vi "nanoVoltRead_Lock-In.vi"() -> ()   [LabVIEW 2014]
uses:
  <vilib>/Utility/file.llb/Write To Spreadsheet File (string).vi
  subvi/Stanford Research 830/Stanford Research 830.lvlib
panel:
  in  "Boolean":bool
  in  "Ref Freq (Hz)":dbl=17.0
  in  "Phase":dbl
  out "Voltage Setpoint (V)":dbl
  in  "VISA resource name":refnum<visa-resource-name>="GPIB0::8::INSTR"
  in  "Time2\n(s)":dbl[](array[numeric])
  in  "Voltage\n(V)":dbl[](array[numeric])
  in  "Filename Label (optional)":string
  in  "Channel\n(0,1,2)":dbl[](array[numeric])
  out "Light Intensity":dbl
  in  "Time1\n(s)":dbl[](array[numeric])
  in  "Intensity\n(0-100%)":dbl[](array[numeric])
  in  "Baud Rate":dbl=57600.0
  in  "Light Port":refnum<visa-resource-name>="COM4"
  in  "Previous Top T":dbl
  in  "Temp Rate (s)":dbl=0.25
  in  "Previous Delta T":dbl
  in  "T read time":dbl
  out "Temp2 (C)":dbl format="%#.4g"
  out "Temp1 (C)":dbl format="%#.4g"
  out "Delta T (C)":dbl format="%#.4g"
  in  "Temp2 Port":tag="Dev2"
  in  "Temp1 Port":tag="Dev1"
  out "Time (s)":dbl caption="Elapsed Time (s)"
  out "XY Graph":cluster{dbl[], dbl[]}[](graph)
  in  "file (use dialog)":path=path "C:/Users/probe_station/Desktop/nanoVolt"
  out "Measurement Number":i32
  in  "stop":bool
  out "Voltage(uV)":dbl
  # "SR830\n2016-01-20\nDavid Ellsworth\nCSU Magnetics Lab"
  # "Ignore These"
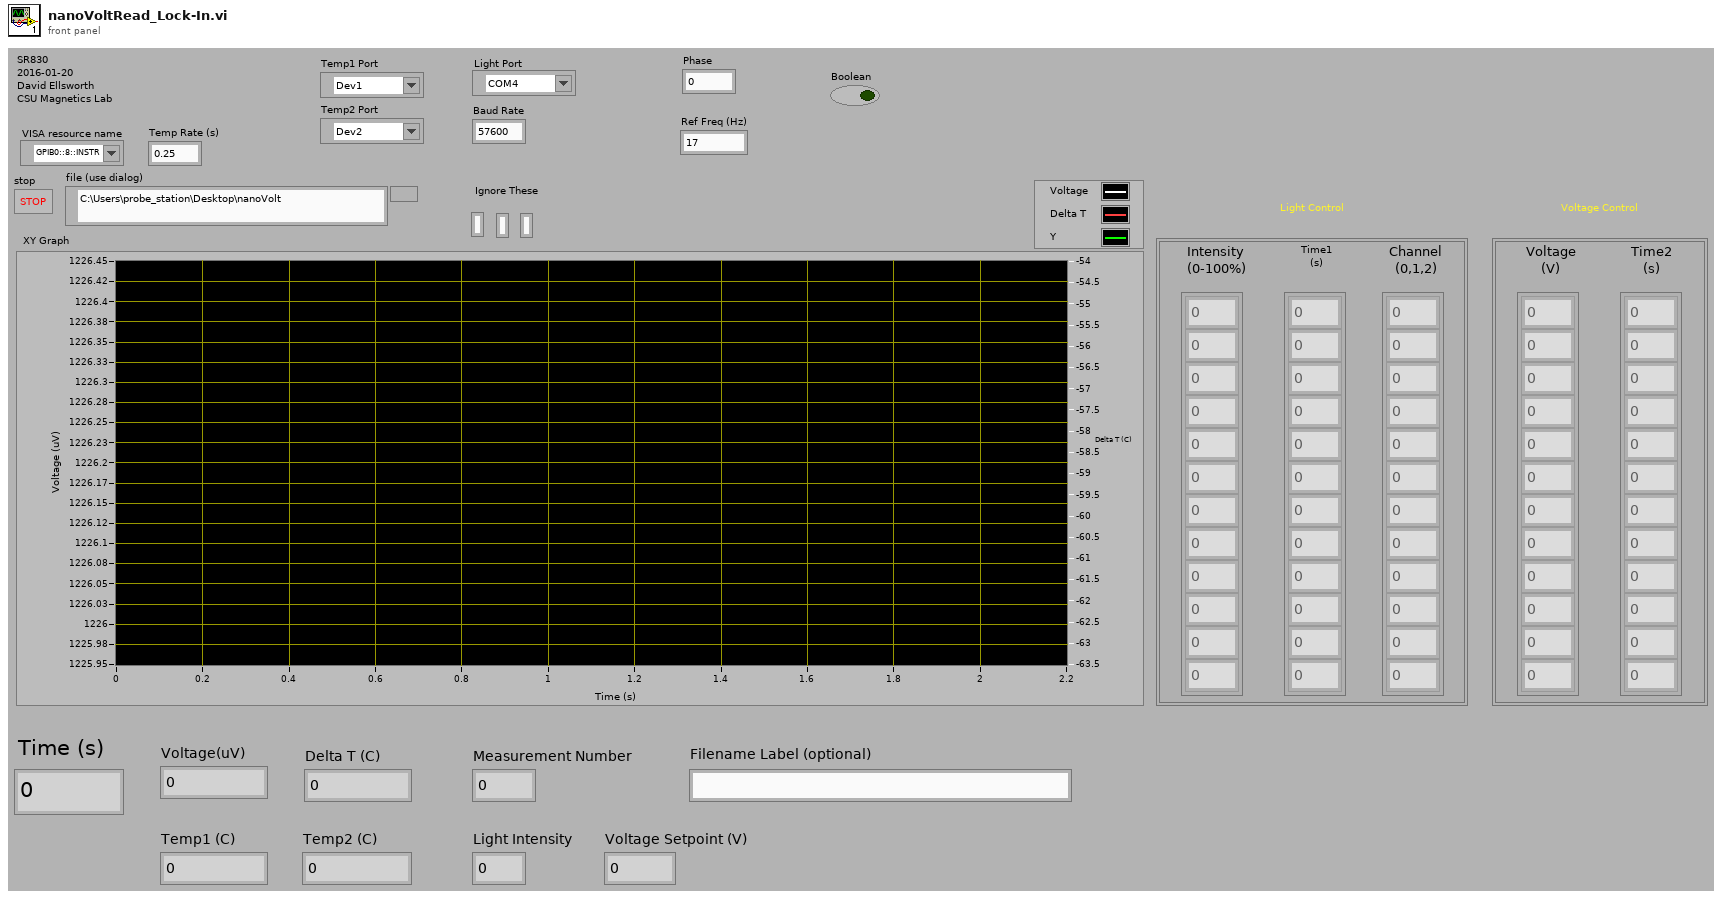
[diagram p1: front panel]
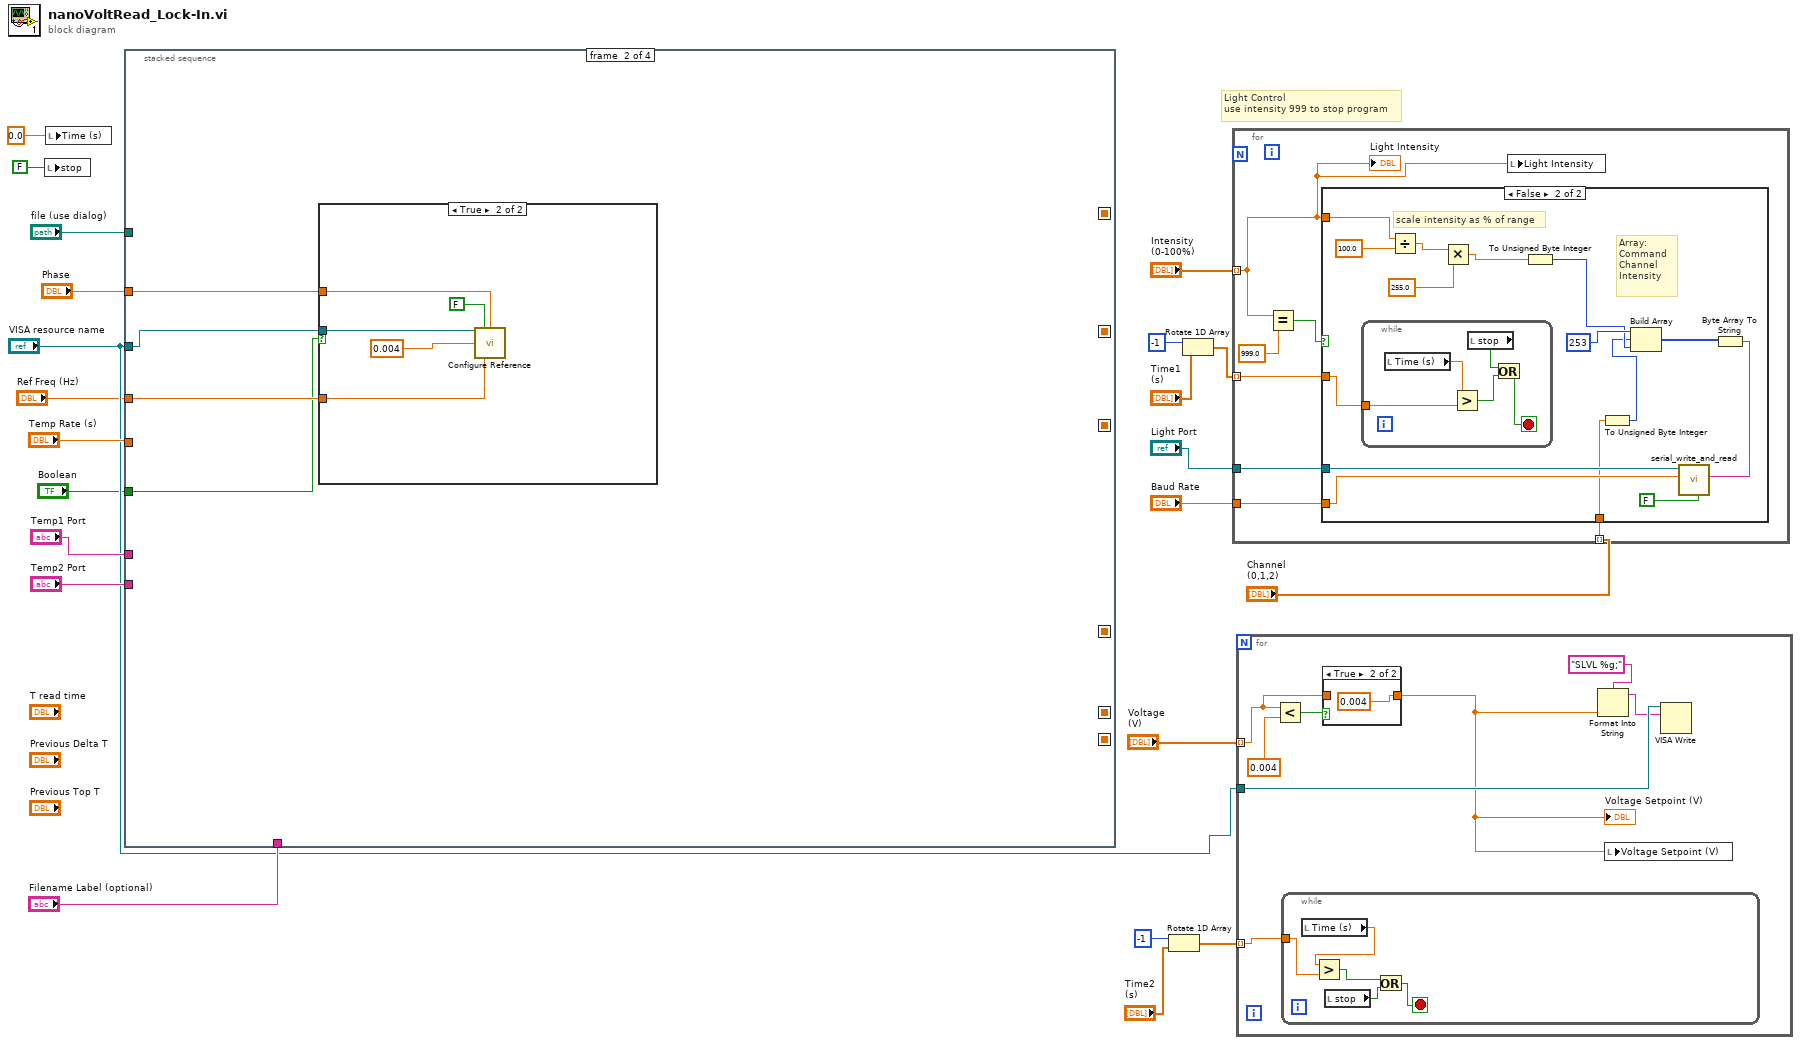
[diagram p0: block diagram]
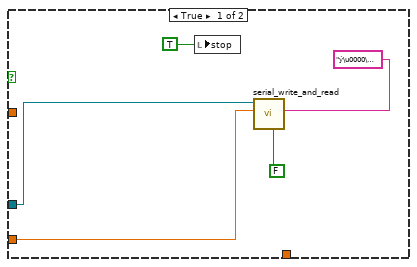
[diagram p3: hidden frame]
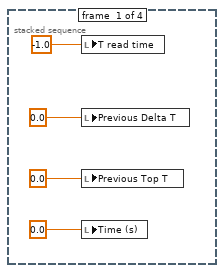
[diagram p4: hidden frame]
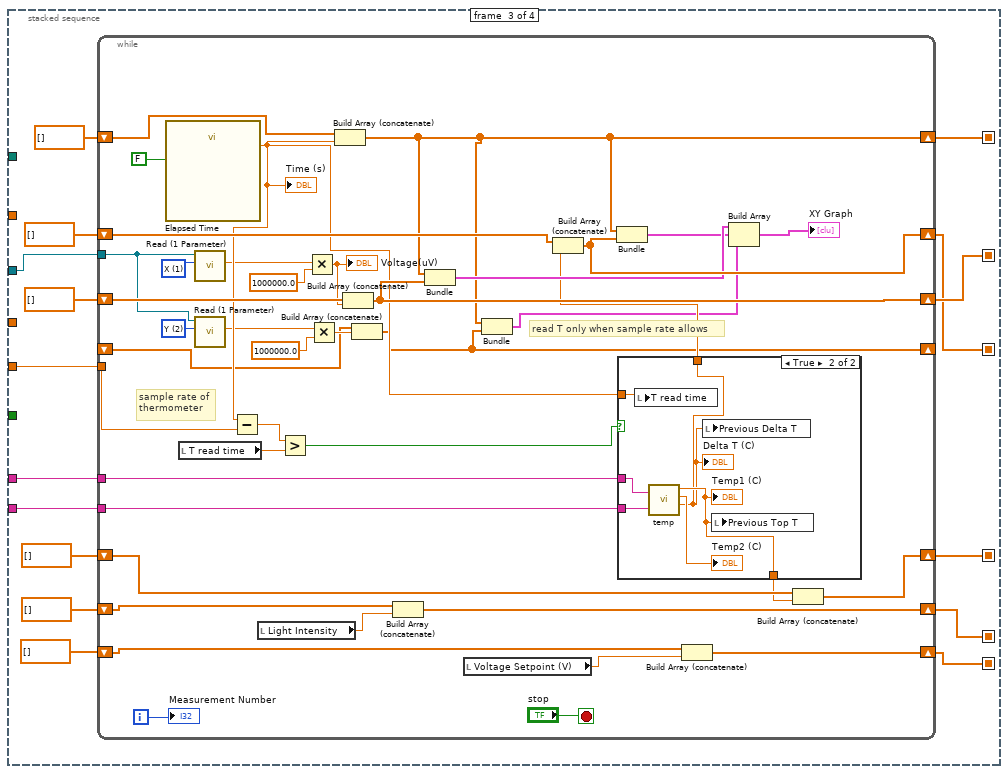
[diagram p6: hidden frame]
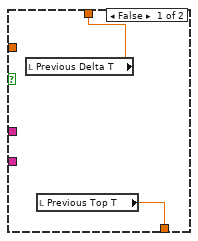
[diagram p7: hidden frame]
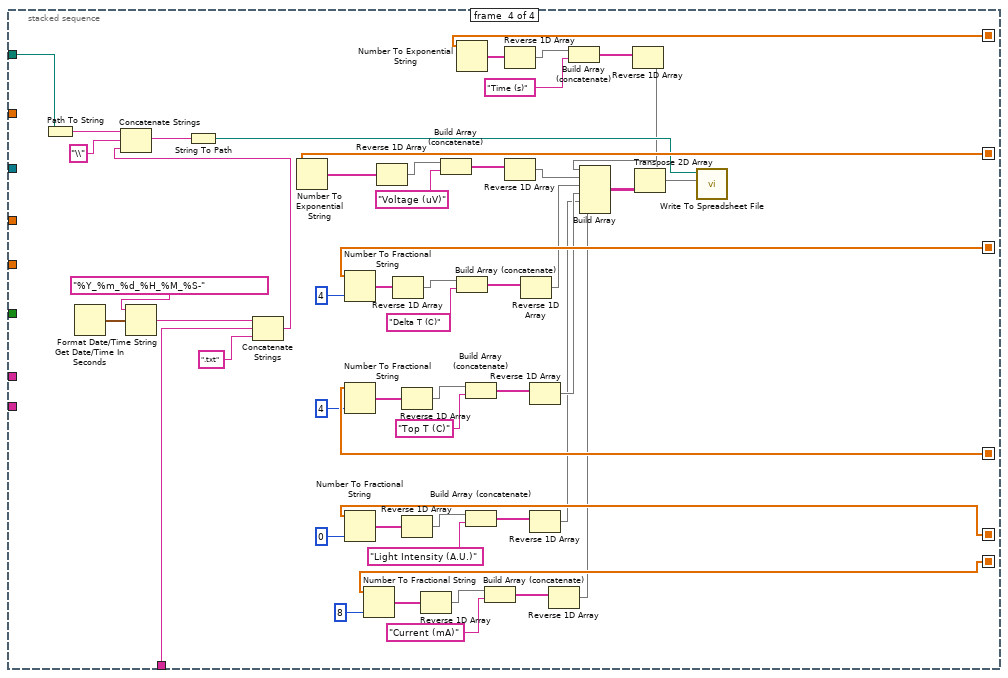
[diagram p8: hidden frame]
diagram:
  # "Light Control\nuse intensity 999 to stop program"
  n1 = local write "stop"(FALSE ("stop")) -> ()
  n2 = local write "Time (s)"(0.0 ("Time (s)")) -> ()
  n3 = stacked-sequence {
    seq-local: [_ _ w50 _] -> [_ _ _ w145]
    seq-local: [_ _ w48 _] -> [_ _ _ w138]
    seq-local: [_ _ w45 _] -> [_ _ _ w142]
    seq-local: [_ _ w42 _] -> [_ _ _ w140]
    seq-local: [_ _ w39 _] -> [_ _ _ w111]
    seq-local: [_ _ w37 _] -> [_ _ _ w102]
    tunnel: "file (use dialog)" -> [_ _ _ w147]
    tunnel: "Temp1 Port" -> [_ _ w47 _]
    tunnel: "Temp2 Port" -> [_ _ w46 _]
    tunnel: "Temp Rate (s)" -> [_ _ w43 _]
    tunnel: "Filename Label (optional)" -> [_ _ _ w108]
    tunnel: "VISA resource name" -> [_ w30 w36 _]
    tunnel: "Phase" -> [_ w29 _ _]
    tunnel: "Ref Freq (Hz)" -> [_ w28 _ _]
    tunnel: "Boolean" -> [_ w27 _ _]
    frame #0 {
      n4 = local write "T read time"(-1.0 ("read T")) -> ()
      n5 = local write "Previous Delta T"(0.0 ("Previous T")) -> ()
      n6 = local write "Previous Top T"(0.0 ("Previous Top T")) -> ()
      n7 = local write "Time (s)"(0.0 ("Time (s)")) -> ()
    }
    frame #1 {
      n8 = case shown="True" w27 {
        tunnel: w30 -> [_ w35]
        tunnel: w29 -> [_ w32]
        tunnel: w28 -> [_ w31]
        frame False {
        }
        frame True {
          n9 = call "Configure Reference.vi"("VISA resource name"=w35, "Auto Phase (T: Enabled)"=FALSE, "Manual Phase (0 Degree)"=w32, "Sine Output Amplitude (1 V)"=0.004, "Internal Reference Frequency (1000 Hz)"=w31) -> ()  [unwired: 9 in, 2 out]
        }
      }
    }
    frame #2 {
      n10 = while {
        shift-right: [w91] -> w50
        shift-left: dbl[] [] -> [w90]
        shift-right: [w54] -> w48
        shift-left: dbl[] [] -> [w88]
        tunnel: w47 -> [w87]
        tunnel: w46 -> [w86]
        shift-right: [w85] -> w45
        shift-left: dbl[] [] -> [w84]
        tunnel: w43 -> [w83]
        shift-right: [w81] -> w42
        shift-left: dbl[] [] -> [w82]
        shift-right: [w79] -> w39
        shift-left: dbl[] [] -> [w80]
        shift-right: [w77] -> w37
        shift-left: dbl[] [] -> [w78]
        tunnel: w36 -> [w59]
        shift-right: [w53] -> _
        shift-left: _ -> [w55]
        i -> [w89]
        stop <- "stop" stop-if-true
        w60 = u16 2 items=["X"=1, "Y"=2, "R"=3, "Theta"=4, "Channel 1"=5, "Channel 2"=6, "Aux In 1"=7, "Aux In 2"=8, "Aux In 3"=9, "Aux In 4"=10] ("Parameter (1: X)")
        w63 = u16 1 items=["X"=1, "Y"=2, "R"=3, "Theta"=4, "Channel 1"=5, "Channel 2"=6, "Aux In 1"=7, "Aux In 2"=8, "Aux In 3"=9, "Aux In 4"=10] ("Parameter (1: X)")
        # "read T only when sample rate allows"
        # "sample rate of\nthermometer"
        n11 = call "Elapsed Time"("Auto Reset"=FALSE) -> ("Elapsed Time (s)"=w70:dbl)  [unwired: 11 in, 7 out]
        "Time (s)" <- w70
        n12 = local read "T read time"() -> (w68:dbl)
        n13 = call "Read (1 Parameter).vi"("Parameter (1: X)"=w63, "VISA resource name"=w59) -> ("Measurement"=w62:dbl)  [unwired: 7 in, 2 out]
        n14 = call "Read (1 Parameter).vi"("Parameter (1: X)"=w60, "VISA resource name"=w59) -> ("Measurement"=w58:dbl)  [unwired: 7 in, 2 out]
        n15 = Subtract(x=w70, y=w83) -> (x-y=w69:dbl)
        n16 = local read "Light Intensity"() -> (w66:dbl)
        n17 = Greater?(x=w69, y=w68) -> (0:w71:bool)
        n18 = Multiply(x=w62, y=1000000.0) -> (x*y=w64:dbl)
        "Voltage(uV)" <- w64
        n19 = Multiply(x=w58, y=1000000.0) -> (x*y=w56:dbl)
        n20 = Build Array (concatenate)(w88, w70) -> (w54:dbl[])
        n21 = Build Array (concatenate)(w90, w64) -> (w91:dbl[])
        n22 = Build Array (concatenate)(w55, w56) -> (w53:dbl[])
        n23 = Build Array (concatenate)(w80, w66) -> (w79:dbl[])
        n24 = Bundle(w54, w91) -> (w75:cluster{dbl[], dbl[]})  [unwired: 1 in]
        n25 = local read "Voltage Setpoint (V)"() -> (w61:dbl)
        n26 = Bundle(w54, w53) -> (w52:cluster{dbl[], dbl[]})  [unwired: 1 in]
        n27 = case shown="True" w71 {
          tunnel: w87 -> [_ w99]
          tunnel: w86 -> [_ w98]
          tunnel: [w94 w95] -> w74
          tunnel: w70 -> [_ w100]
          tunnel: [w93 w97] -> w67
          frame False {
            n28 = local read "Previous Delta T"() -> (w94:dbl)
            n29 = local read "Previous Top T"() -> (w93:dbl)
          }
          frame True {
            n30 = local write "T read time"(w100) -> ()
            n31 = call "temp.vi"("Temp2 (Bottom) Port"=w98, "Temp1 (Top) Port"=w99) -> ("Delta T"=w95:dbl, "Bottom"=→"Temp2 (C)":dbl, "Top"=w97:dbl)  [unwired: 2 out]
            "Delta T (C)" <- w95
            "Temp1 (C)" <- w97
            n32 = local write "Previous Delta T"(w95) -> ()
            n33 = local write "Previous Top T"(w97) -> ()
          }
        }
        n34 = Build Array (concatenate)(w84, w74) -> (w85:dbl[])
        n35 = Bundle(w54, w85) -> (w72:cluster{dbl[], dbl[]})  [unwired: 1 in]
        n36 = Build Array (concatenate)(w78, w61) -> (w77:dbl[])
        n37 = Build Array(w75, w72, w52) -> (→"XY Graph":cluster{dbl[], dbl[]}[])
        n38 = Build Array (concatenate)(w82, w67) -> (w81:dbl[])
        "Measurement Number" <- w89
      }
    }
    frame #3 {
      n39 = Path To String(path=w147) -> (string=w150:string)
      n40 = Get Date/Time In Seconds() -> (seconds since 1Jan1904=w153:timestamp)
      n41 = Format Date/Time String(time format string (%c)="%Y_%m_%d_%H_%M_%S-", seconds (now)=w153) -> (date/time string=w151:string)  [unwired: 1 in]
      n42 = Concatenate Strings(w151, w108, ".txt" ("string")) -> (w146:string)
      n43 = Concatenate Strings(w150, "\\" ("string"), w146) -> (w148:string)
      n44 = String To Path(string=w148) -> (path=w144:path)
      n45 = Number To Exponential String(number=w145) -> (E-format string=w132:string[])  [unwired: 3 in]
      n46 = Number To Fractional String(number=w142, precision (6)=i16 4) -> (F-format string=w127:string[])  [unwired: 2 in]
      n47 = Number To Fractional String(number=w140, precision (6)=i16 4) -> (F-format string=w120:string[])  [unwired: 2 in]
      n48 = Number To Fractional String(number=w111, precision (6)=i16 0) -> (F-format string=w112:string[])  [unwired: 2 in]
      n49 = Number To Fractional String(number=w102, precision (6)=i16 8) -> (F-format string=w103:string[])  [unwired: 2 in]
      n50 = Reverse 1D Array(array=w132) -> (reversed array=w131:string[])
      n51 = Reverse 1D Array(array=w127) -> (reversed array=w126:string[])
      n52 = Reverse 1D Array(array=w120) -> (reversed array=w122:string[])
      n53 = Reverse 1D Array(array=w112) -> (reversed array=w114:string[])
      n54 = Reverse 1D Array(array=w103) -> (reversed array=w105:string[])
      n55 = Build Array (concatenate)(w131, "Voltage (uV)") -> (w130:string[])
      n56 = Number To Exponential String(number=w138) -> (E-format string=w136:string[])  [unwired: 3 in]
      n57 = Build Array (concatenate)(w126, "Delta T (C)") -> (w128:string[])
      n58 = Build Array (concatenate)(w122, "Top T (C)") -> (w123:string[])
      n59 = Build Array (concatenate)(w114, "Light Intensity (A.U.)") -> (w115:string[])
      n60 = Build Array (concatenate)(w105, "Current (mA)") -> (w106:string[])
      n61 = Reverse 1D Array(array=w136) -> (reversed array=w135:string[])
      n62 = Reverse 1D Array(array=w130) -> (reversed array=w129:string[])
      n63 = Reverse 1D Array(array=w128) -> (reversed array=w125:string[])
      n64 = Reverse 1D Array(array=w123) -> (reversed array=w119:string[])
      n65 = Reverse 1D Array(array=w115) -> (reversed array=w110:string[])
      n66 = Reverse 1D Array(array=w106) -> (reversed array=w101:string[])
      n67 = Build Array (concatenate)(w135, "Time (s)") -> (w134:string[])
      n68 = Reverse 1D Array(array=w134) -> (reversed array=w133:string[])
      n69 = Build Array(w133, w129, w125, w119, w110, w101) -> (w137:string[][])
      n70 = Transpose 2D Array(2D array=w137) -> (transposed array=w143:string[][])
      n71 = call-poly <vilib>:"Write To Spreadsheet File.vi"("2D data"=w143, "file path (dialog if empty)"=w144) -> ()  [unwired: 6 in, 1 out]
    }
  }
  n72 = Rotate 1D Array(1:"Time2\n(s)", 2:-1 ("n")) -> (0:w5:dbl[])
  n73 = Rotate 1D Array(1:"Time1\n(s)", 2:-1 ("n")) -> (0:w11:dbl[])
  n74 = for {
    tunnel: "Intensity\n(0-100%)" -> [w154] mode=indexing
    tunnel: w11 -> [w158] mode=indexing
    tunnel: "Light Port" -> [w160]
    tunnel: "Baud Rate" -> [w159]
    tunnel: "Channel\n(0,1,2)" -> [w155] mode=indexing
    n75 = Equal?(x=w154, y=999.0) -> (x = y?=w157:bool)
    n76 = case shown="False" w157 {
      tunnel: w160 -> [w164 w172]
      tunnel: w159 -> [w163 w171]
      tunnel: w158 -> [_ w170]
      tunnel: w154 -> [_ w169]
      tunnel: w155 -> [_ w167]
      frame True {
        n77 = local write "stop"(TRUE ("stop")) -> ()
        n78 = call "serial_write_and_read.vi"("VISA resource name"=w164, "baud rate"=w163, "read"=FALSE, "string to write"="ý\u0000\u0000") -> ()  [unwired: 6 in, 1 out]
      }
      frame False {
        # "Array:\nCommand\nChannel\nIntensity"
        # "scale intensity as % of range"
        n79 = while {
          tunnel: w170 -> [w182]
          stop <- w185 stop-if-true
          n80 = local read "Time (s)"() -> (w183:dbl)
          n81 = Greater?(x=w183, y=w182) -> (0:w181:bool)
          n82 = local read "stop"() -> (w184:bool)
          n83 = Or(x=w184, y=w181) -> (x .or. y?=w185:bool)
        }
        n84 = Divide(x=w169, y=100.0) -> (x/y=w179:dbl)
        n85 = Multiply(x=w179, y=255.0) -> (x*y=w177:dbl)
        n86 = To Unsigned Byte Integer(number=w177) -> (unsigned 8bit integer=w168:u8)
        n87 = To Unsigned Byte Integer(number=w167) -> (unsigned 8bit integer=w166:u8)
        n88 = Build Array(u8 253 ("element"), w166, w168) -> (w175:u8[])
        n89 = Byte Array To String(unsigned byte array=w175) -> (string=w174:string)
        n90 = call "serial_write_and_read.vi"("VISA resource name"=w172, "baud rate"=w171, "read"=FALSE, "string to write"=w174) -> ()  [unwired: 6 in, 1 out]
      }
    }
    n91 = local write "Light Intensity"(w154) -> ()
    "Light Intensity" <- w154
  }
  n92 = for {
    tunnel: "Voltage\n(V)" -> [w187] mode=indexing
    tunnel: w5 -> [w193] mode=indexing
    tunnel: "VISA resource name" -> [w192]
    n93 = Less?(x=w187, y=0.004) -> (x < y?=w188:bool)
    n94 = while {
      tunnel: w193 -> [w199]
      stop <- w200 stop-if-true
      n95 = local read "Time (s)"() -> (w198:dbl)
      n96 = Greater?(x=w198, y=w199) -> (0:w196:bool)
      n97 = local read "stop"() -> (w197:bool)
      n98 = Or(x=w196, y=w197) -> (x .or. y?=w200:bool)
    }
    n99 = case shown="True" w188 {
      tunnel: w187 -> [w194 _]
      tunnel: [w194 0.004 ("Numeric")] -> w186
      frame False {
      }
      frame True {
      }
    }
    "Voltage Setpoint (V)" <- w186
    n100 = Format Into String(format string="SLVL %g;", w186) -> (resulting string=w190:string)  [unwired: 2 in, 1 out]
    n101 = local write "Voltage Setpoint (V)"(w186) -> ()
    n102 = VISA Write(VISA resource name=w192, write buffer=w190) -> ()  [unwired: 1 in, 3 out]
  }
